vi "Untitled 3.vi"(6 "Waveform Chart":dbl(graph), 8 "Numeric 4":dbl, 9 "Numeric 3":dbl, 10 "Numeric 2":dbl, 11 "Numeric":dbl) -> (1 "Numeric 5":dbl, 2 "Numeric 6":dbl)   [LabVIEW 2025, in "MCP Server.lvlib"]
uses:
  MCP Server.lvlib
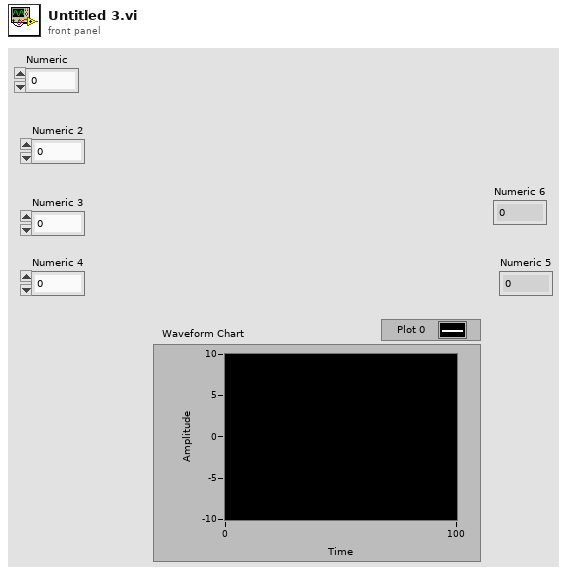
[diagram p1: front panel]
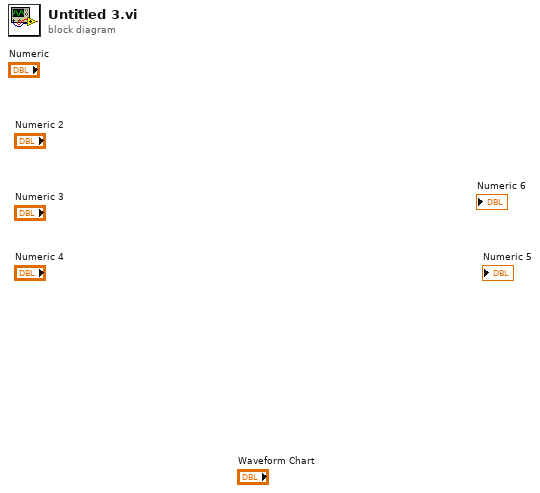
[diagram p0: block diagram]
diagram:
